vi "Initialize.vi"(8 "error in (no error)":errorcluster, 10 "VI Refnum":refnum<vi>, 11 "Warning Dialog in":refnum<class "Warning Dialog.lvclass">) -> (0 "error out":errorcluster, 3 "Warning Dialog out":refnum<class "Warning Dialog.lvclass">)   [LabVIEW 2015, in "Warning Dialog.lvclass"]
doc: "<b> </b> <b> </b>\n©2016 Q Software Innovations, LLC (QSI)\nwritten by Quentin Alldredge\nproduced in LabVIEW 2015\n\nsupport@qsoftwareinnovations.com\nwww.qsoftwareinnovations.com\n\nAll rights reserved.\n\nRedistribution and use in source and binary forms, with or without modification, are permitted provided that the following conditions are met:\n\n * Redistributions of source code must retain the above copyright notice, this list of conditions and the following disclaimer.\n * Redistributions in binary form must reproduce the above copyright notice, this list of conditions and the following disclaimer in the documentation and/or other materials provided with the distribution.\n * Neither the name of Q Software Innovations, LLC. nor the names of its contributors may be used to endorse or promote products derived from this software without specific prior written permission.\n\nTHIS SOFTWARE IS PROVIDED BY THE COPYRIGHT HOLDERS AND CONTRIBUTORS \"AS IS\" AND ANY EXPRESS OR IMPLIED WARRANTIES, INCLUDING, BUT NOT LIMITED TO, THE IMPLIED WARRANTIES OF MERCHANTABILITY AND FITNESS FOR A PARTICULAR PURPOSE ARE DISCLAIMED. IN NO EVENT SHALL THE COPYRIGHT OWNER OR CONTRIBUTORS BE LIABLE FOR ANY DIRECT, INDIRECT, INCIDENTAL, SPECIAL, EXEMPLARY, OR CONSEQUENTIAL DAMAGES (INCLUDING, BUT NOT LIMITED TO, PROCUREMENT OF SUBSTITUTE GOODS OR SERVICES; LOSS OF USE, DATA, OR PROFITS; OR BUSINESS INTERRUPTION) HOWEVER CAUSED AND ON ANY THEORY OF LIABILITY, WHETHER IN CONTRACT, STRICT LIABILITY, OR TORT (INCLUDING NEGLIGENCE OR OTHERWISE) ARISING IN ANY WAY OUT OF THE USE OF THIS SOFTWARE, EVEN IF ADVISED OF THE POSSIBILITY OF SUCH DAMAGE."
uses:
  Warning Dialog.lvclass
  Dialog/Dialog.lvclass
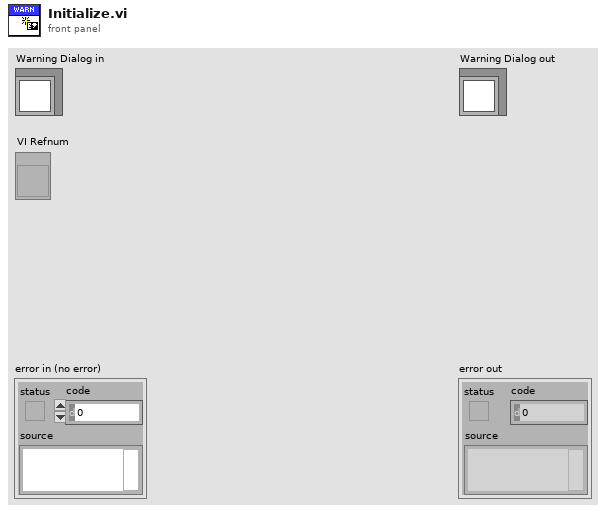
[diagram p1: front panel]
types:
  T1 = enum32{"Invalid", "Standard", "Closed", "Hidden", "Minimized", "Maximized"}
  T2 = enum32{"Invalid", "Default", "Floating", "Floating/Auto-Hide", "Modal"}
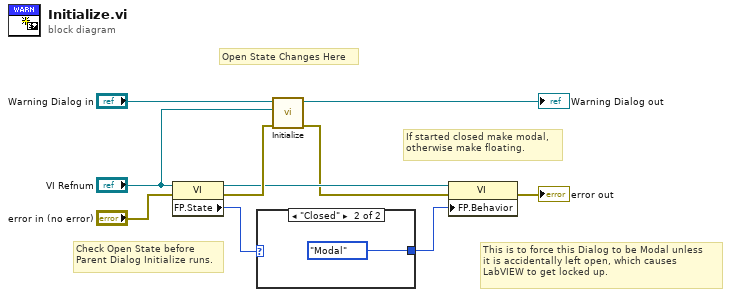
[diagram p0: block diagram]
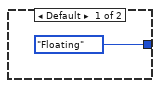
[diagram p2: hidden frame]
diagram:
  # "Check Open State before\nParent Dialog Initialize runs."
  # "Open State Changes Here"
  # "This is to force this Dialog to be Modal unless\nit is accidentally left open, which causes \nLabVIEW to get locked up."
  # "If started closed make modal,\notherwise make floating."
  n1 = property class="VI"(reference="VI Refnum", error in="error in (no error)") -> (reference out=w5:refnum<vi>, error out=w7:errorcluster, "FP.State"=w2:T1)
  n2 = case shown="\"Closed\"" w2 {
    tunnel: [T2."Floating" ("Front Panel Window:Behavior") T2."Modal" ("Front Panel Window:Behavior")] -> w1
    frame Default {
    }
    frame "Closed" {
    }
  }
  n3 = call-parent "Initialize.vi"("error in (no error)"=w7, "VI Refnum"="VI Refnum", "Dialog in"="Warning Dialog in") -> ("error out"=w4:errorcluster, "Dialog out"=→"Warning Dialog out":refnum<class "Warning Dialog.lvclass">)  [unwired: 7 in]
  n4 = property class="VI"(reference=w5, error in=w4, "FP.Behavior"=w1) -> (error out=→"error out":errorcluster)  [unwired: 1 out]
